vi "Auton_S2_Right_Switch.vi"   [LabVIEW 2017]
uses:
  <vilib>/Rock Robotics/WPI/Utilities/WPI_GetSetVariantRefNum.vi
  Robot Global Data.vi
  <vilib>/Rock Robotics/WPI/RobotDrive/WPI_RobotDriveArcadeDrive_Standard(NoSaturation).vi
types:
  T1 = typedef "WPI_RobotDriveDevRef.ctl" = cluster{"DevStatus":errorcluster, "Motors[]":T2[], "Square Inputs":bool, "Max Output":dbl}
  T2 = typedef "WPI_MotorControlDeviceRef.ctl" = cluster{"DeviceStatus":errorcluster, "Type":T3, "PWM":cluster{"PWM Channel":T4, "DeadBand":T5}, "CAN":cluster{"Device Number":u8, "SetOutput VI Ref":variant, "GetOutput VI Ref":variant, "Enable VI Ref":variant, "Disable VI Ref":variant, "Data":variant}, "Invert":bool, "DIO PWM":cluster{"PWM \"Enable\" Channel":T4, "DIOChannel":T6, "PWM Rate":dbl}}
  T3 = typedef "WPI_MotorControlType.ctl" = enum16{"PWM", "CAN", "DIO PWM"}
  T4 = typedef "FPGA_DIOPWMChannel.ctl" = enum8{"PWM 0", "PWM 1", "PWM 2", "PWM 3", "PWM 4", "PWM 5", "PWM 6", "PWM 7", "PWM 8", "PWM 9", "PWM MXP 0", "PWM MXP 1", "PWM MXP 2", "PWM MXP 3", "PWM MXP 4", "PWM MXP 5", "PWM MXP 6", "PWM MXP 7", "PWM MXP 8", "PWM MXP 9", "Invalid"}
  T5 = typedef "WPI_PWMDeadband.ctl" = cluster{"Name":string, "maxPositivePwm":i32, "minPositivePwm":i32, "centerPwm":i32, "maxNegativePwm":i32, "minNegativePwm":i32, "angularRange":u16}
  T6 = typedef "FPGA_DIOChannel.ctl" = enum8{"DIO 0", "DIO 1", "DIO 2", "DIO 3", "DIO 4", "DIO 5", "DIO 6", "DIO 7", "DIO 8", "DIO 9", "DIO MXP 0", "DIO MXP 1", "DIO MXP 2", "DIO MXP 3", "DIO MXP 4", "DIO MXP 5", "DIO MXP 6", "DIO MXP 7", "DIO MXP 8", "DIO MXP 9", "DIO MXP 10", "DIO MXP 11", "DIO MXP 12", "DIO MXP 13", "DIO MXP 14", "DIO MXP 15", "SPI Port CS1", "SPI Port CS2", "SPI Port CS3", "SPI Port MISO", "SPI Port MOSI", "Invalid"}
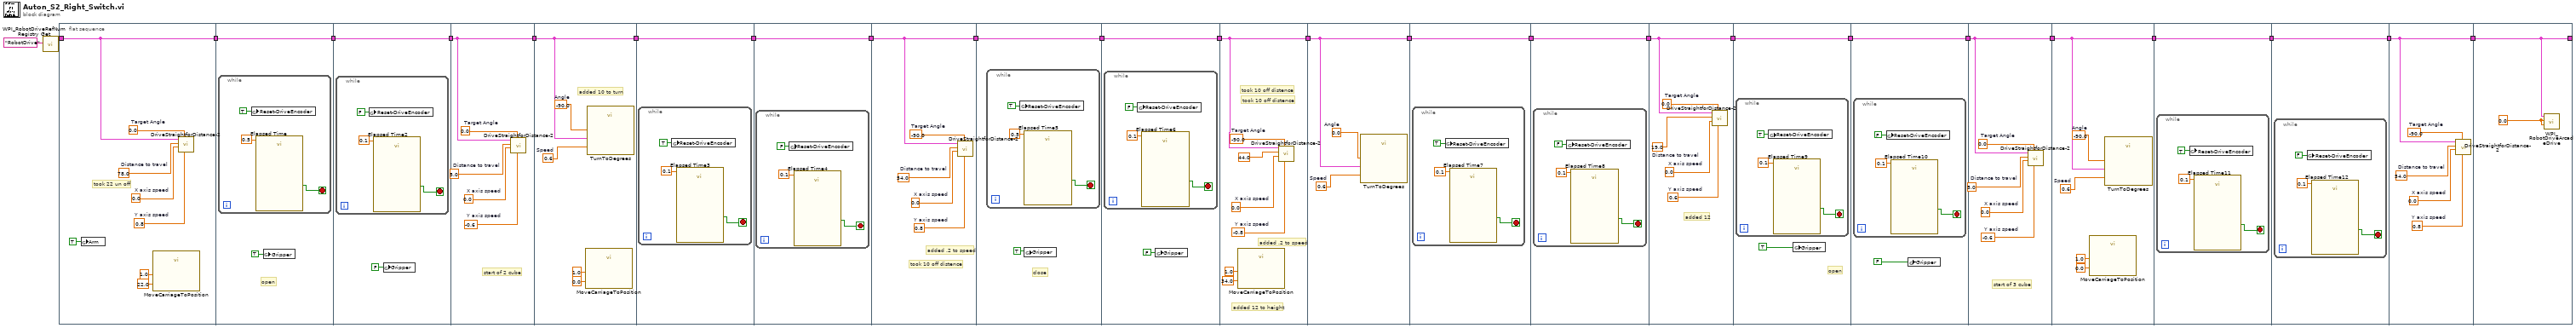
[diagram p0: block diagram]
diagram:
  n1 = call <vilib>:"WPI_RobotDriveRefNum Registry Get.vi"("refnum name"="RobotDrive") -> ("RobotDriveDevRef"=w23:T1)  [unwired: 9 in, 1 out]
  n2 = flat-sequence {
    tunnel: [w32] -> w22
    tunnel: w23 -> [w32]
    tunnel: w22 -> [w34]
    tunnel: [w34] -> w21
    tunnel: w21 -> [w39]
    tunnel: [w39] -> w20
    tunnel: w20 -> [w43]
    tunnel: [w43] -> w19
    tunnel: w19 -> [w50]
    tunnel: [w50] -> w18
    tunnel: w18 -> [w53]
    tunnel: [w53] -> w17
    tunnel: w17 -> [w57]
    tunnel: [w57] -> w16
    tunnel: w16 -> [w61]
    tunnel: [w61] -> w15
    tunnel: w15 -> [w67]
    tunnel: [w67] -> w14
    tunnel: w14 -> [w72]
    tunnel: [w72] -> w13
    tunnel: w13 -> [w78]
    tunnel: [w78] -> w12
    tunnel: w12 -> [w83]
    tunnel: [w83] -> w11
    tunnel: w11 -> [w86]
    tunnel: [w86] -> w10
    tunnel: w10 -> [w90]
    tunnel: [w90] -> w9
    tunnel: w9 -> [w94]
    tunnel: [w94] -> w8
    tunnel: w8 -> [w100]
    tunnel: [w100] -> w7
    tunnel: w7 -> [w105]
    tunnel: [w105] -> w6
    tunnel: w6 -> [w109]
    tunnel: [w109] -> w5
    tunnel: w5 -> [w114]
    tunnel: [w114] -> w4
    tunnel: w4 -> [w119]
    tunnel: [w119] -> w3
    tunnel: w3 -> [w123]
    tunnel: [w123] -> w2
    tunnel: w2 -> [w127]
    tunnel: [w127] -> w1
    tunnel: [w132] -> _
    tunnel: w1 -> [w132]
    frame #0 {
      w28 = 0.0  # Target Angle
      w29 = 0.8  # Y axis speed
      w30 = 0.0  # X axis speed
      w31 = 78.0  # Distance to travel
      # "took 22 un off"
      n3 = global write "Robot Global Data.vi" "Arm"(TRUE ("Arm")) -> ()
      n4 = call "MoveCarriageToPosition.vi"("Lift Speed"=1.0, "Target Height"=22.0) -> ()  [unwired: 10 in]
      n5 = call "DriveStraightforDistance-2.vi"("Y axis speed"=w29, "Target Angle"=w28, "X axis speed"=w30, "Distance to travel"=w31, "RobotDriveDevRef"=w32) -> ()  [unwired: 7 in]
    }
    frame #1 {
      # "open"
      n6 = while {
        stop <- w37 stop-if-true
        n7 = global write "Robot Global Data.vi" "Reset-DriveEncoder"(TRUE ("Reset-DriveEncoder")) -> ()
        n8 = call "Elapsed Time"("Time Target (s)"=0.5) -> ("Time has Elapsed"=w37:bool)  [unwired: 11 in, 7 out]
      }
      n9 = global write "Robot Global Data.vi" "Gripper"(TRUE ("Gripper")) -> ()
    }
    frame #2 {
      n10 = while {
        stop <- w42 stop-if-true
        n11 = global write "Robot Global Data.vi" "Reset-DriveEncoder"(FALSE ("Reset-DriveEncoder")) -> ()
        n12 = call "Elapsed Time2"("Time Target (s)"=0.1) -> ("Time has Elapsed"=w42:bool)  [unwired: 11 in, 7 out]
      }
      n13 = global write "Robot Global Data.vi" "Gripper"(FALSE ("Gripper")) -> ()
    }
    frame #3 {
      w44 = 0.0  # Target Angle
      w45 = -0.6  # Y axis speed
      w46 = 0.0  # X axis speed
      w47 = 5.0  # Distance to travel
      # "start of 2 cube"
      n14 = call "DriveStraightforDistance-2.vi"("Y axis speed"=w45, "Target Angle"=w44, "X axis speed"=w46, "Distance to travel"=w47, "RobotDriveDevRef"=w43) -> ()  [unwired: 7 in]
    }
    frame #4 {
      w51 = -90.0  # Angle
      w52 = 0.6  # Speed
      # "added 10 to turn"
      n15 = call "MoveCarriageToPosition.vi"("Lift Speed"=1.0, "Target Height"=0.0) -> ()  [unwired: 10 in]
      n16 = call "TurnToDegrees.vi"("Speed"=w52, "RobotDriveDevRef"=w50, "Angle"=w51) -> ()  [unwired: 9 in]
    }
    frame #5 {
      n17 = while {
        stop <- w56 stop-if-true
        n18 = global write "Robot Global Data.vi" "Reset-DriveEncoder"(TRUE ("Reset-DriveEncoder")) -> ()
        n19 = call "Elapsed Time3"("Time Target (s)"=0.1) -> ("Time has Elapsed"=w56:bool)  [unwired: 11 in, 7 out]
      }
    }
    frame #6 {
      n20 = while {
        stop <- w60 stop-if-true
        n21 = global write "Robot Global Data.vi" "Reset-DriveEncoder"(FALSE ("Reset-DriveEncoder")) -> ()
        n22 = call "Elapsed Time4"("Time Target (s)"=0.1) -> ("Time has Elapsed"=w60:bool)  [unwired: 11 in, 7 out]
      }
    }
    frame #7 {
      w62 = -90.0  # Target Angle
      w63 = 0.8  # Y axis speed
      w64 = 0.0  # X axis speed
      w65 = 54.0  # Distance to travel
      # "added .2 to speed"
      # "took 10 off distence"
      n23 = call "DriveStraightforDistance-2.vi"("Y axis speed"=w63, "Target Angle"=w62, "X axis speed"=w64, "Distance to travel"=w65, "RobotDriveDevRef"=w61) -> ()  [unwired: 7 in]
    }
    frame #8 {
      # "close"
      n24 = while {
        stop <- w70 stop-if-true
        n25 = global write "Robot Global Data.vi" "Reset-DriveEncoder"(TRUE ("Reset-DriveEncoder")) -> ()
        n26 = call "Elapsed Time5"("Time Target (s)"=0.5) -> ("Time has Elapsed"=w70:bool)  [unwired: 11 in, 7 out]
      }
      n27 = global write "Robot Global Data.vi" "Gripper"(TRUE ("Gripper")) -> ()
    }
    frame #9 {
      n28 = while {
        stop <- w75 stop-if-true
        n29 = global write "Robot Global Data.vi" "Reset-DriveEncoder"(FALSE ("Reset-DriveEncoder")) -> ()
        n30 = call "Elapsed Time6"("Time Target (s)"=0.1) -> ("Time has Elapsed"=w75:bool)  [unwired: 11 in, 7 out]
      }
      n31 = global write "Robot Global Data.vi" "Gripper"(FALSE ("Gripper")) -> ()
    }
    frame #10 {
      w80 = -90.0  # Target Angle
      w81 = -0.8  # Y axis speed
      w82 = 0.0  # X axis speed
      # "took 10 off distence"
      # "added .2 to speed"
      # "took 10 off distence"
      # "added 12 to height"
      n32 = call "MoveCarriageToPosition.vi"("Lift Speed"=1.0, "Target Height"=34.0) -> ()  [unwired: 10 in]
      n33 = call "DriveStraightforDistance-2.vi"("Y axis speed"=w81, "Target Angle"=w80, "X axis speed"=w82, "Distance to travel"=44.0, "RobotDriveDevRef"=w78) -> ()  [unwired: 7 in]
    }
    frame #11 {
      w84 = 0.0  # Angle
      w85 = 0.6  # Speed
      n34 = call "TurnToDegrees.vi"("Speed"=w85, "RobotDriveDevRef"=w83, "Angle"=w84) -> ()  [unwired: 9 in]
    }
    frame #12 {
      n35 = while {
        stop <- w89 stop-if-true
        n36 = global write "Robot Global Data.vi" "Reset-DriveEncoder"(TRUE ("Reset-DriveEncoder")) -> ()
        n37 = call "Elapsed Time7"("Time Target (s)"=0.1) -> ("Time has Elapsed"=w89:bool)  [unwired: 11 in, 7 out]
      }
    }
    frame #13 {
      n38 = while {
        stop <- w93 stop-if-true
        n39 = global write "Robot Global Data.vi" "Reset-DriveEncoder"(FALSE ("Reset-DriveEncoder")) -> ()
        n40 = call "Elapsed Time8"("Time Target (s)"=0.1) -> ("Time has Elapsed"=w93:bool)  [unwired: 11 in, 7 out]
      }
    }
    frame #14 {
      w95 = 0.0  # Target Angle
      w98 = 0.6  # Y axis speed
      w97 = 0.0  # X axis speed
      w96 = 19.0  # Distance to travel
      # "added 12"
      n41 = call "DriveStraightforDistance-2.vi"("Y axis speed"=w98, "Target Angle"=w95, "X axis speed"=w97, "Distance to travel"=w96, "RobotDriveDevRef"=w94) -> ()  [unwired: 7 in]
    }
    frame #15 {
      # "open"
      n42 = while {
        stop <- w103 stop-if-true
        n43 = global write "Robot Global Data.vi" "Reset-DriveEncoder"(TRUE ("Reset-DriveEncoder")) -> ()
        n44 = call "Elapsed Time9"("Time Target (s)"=0.1) -> ("Time has Elapsed"=w103:bool)  [unwired: 11 in, 7 out]
      }
      n45 = global write "Robot Global Data.vi" "Gripper"(TRUE ("Gripper")) -> ()
    }
    frame #16 {
      n46 = while {
        stop <- w108 stop-if-true
        n47 = global write "Robot Global Data.vi" "Reset-DriveEncoder"(FALSE ("Reset-DriveEncoder")) -> ()
        n48 = call "Elapsed Time10"("Time Target (s)"=0.1) -> ("Time has Elapsed"=w108:bool)  [unwired: 11 in, 7 out]
      }
      n49 = global write "Robot Global Data.vi" "Gripper"(FALSE ("Gripper")) -> ()
    }
    frame #17 {
      w110 = 0.0  # Target Angle
      w111 = -0.6  # Y axis speed
      w112 = 0.0  # X axis speed
      w113 = 5.0  # Distance to travel
      # "start of 3 cube"
      n50 = call "DriveStraightforDistance-2.vi"("Y axis speed"=w111, "Target Angle"=w110, "X axis speed"=w112, "Distance to travel"=w113, "RobotDriveDevRef"=w109) -> ()  [unwired: 7 in]
    }
    frame #18 {
      w117 = -90.0  # Angle
      w118 = 0.6  # Speed
      n51 = call "MoveCarriageToPosition.vi"("Lift Speed"=1.0, "Target Height"=0.0) -> ()  [unwired: 10 in]
      n52 = call "TurnToDegrees.vi"("Speed"=w118, "RobotDriveDevRef"=w114, "Angle"=w117) -> ()  [unwired: 9 in]
    }
    frame #19 {
      n53 = while {
        stop <- w122 stop-if-true
        n54 = global write "Robot Global Data.vi" "Reset-DriveEncoder"(TRUE ("Reset-DriveEncoder")) -> ()
        n55 = call "Elapsed Time11"("Time Target (s)"=0.1) -> ("Time has Elapsed"=w122:bool)  [unwired: 11 in, 7 out]
      }
    }
    frame #20 {
      n56 = while {
        stop <- w126 stop-if-true
        n57 = global write "Robot Global Data.vi" "Reset-DriveEncoder"(FALSE ("Reset-DriveEncoder")) -> ()
        n58 = call "Elapsed Time12"("Time Target (s)"=0.1) -> ("Time has Elapsed"=w126:bool)  [unwired: 11 in, 7 out]
      }
    }
    frame #21 {
      w128 = -90.0  # Target Angle
      w129 = 0.8  # Y axis speed
      w130 = 0.0  # X axis speed
      w131 = 54.0  # Distance to travel
      n59 = call "DriveStraightforDistance-2.vi"("Y axis speed"=w129, "Target Angle"=w128, "X axis speed"=w130, "Distance to travel"=w131, "RobotDriveDevRef"=w127) -> ()  [unwired: 7 in]
    }
    frame #22 {
      w133 = 0.0 ("X axis value")
      n60 = call-poly <vilib>:"WPI_RobotDriveArcadeDrive.vi"("Y axis value"=w133, "X axis value"=w133, "RobotDriveDevRef"=w132) -> ()  [unwired: 6 in, 3 out]
    }
  }
